vi "Initialize Parameter File.vi"(6 "File type":enum16{"INI"}(ring), 8 "error in (no error)":errorcluster, 9 "create file if necessary (T)":bool=TRUE, 10 "configuration file path (blank opens dialog)":path, 11 "CD Parameter Manager in":refnum<class "CD Parameter Manager.lvclass">) -> (0 "error out":errorcluster, 3 "CD Parameter Manager out":refnum<class "CD Parameter Manager.lvclass">)   [LabVIEW 2019, in "CD Parameter Manager API.lvlib" / "CD Parameter Manager.lvclass"]
uses:
  CD Parameter Manager.lvclass
  Parameter INI File/Parameter INI File.lvclass
  C:/Repositories/UI-Control-Initializer-API/Source/Parameter Generic File/Parameter Generic File.lvclass
  CD Parameter Manager.lvclass/CD Parameter Manager.ctl
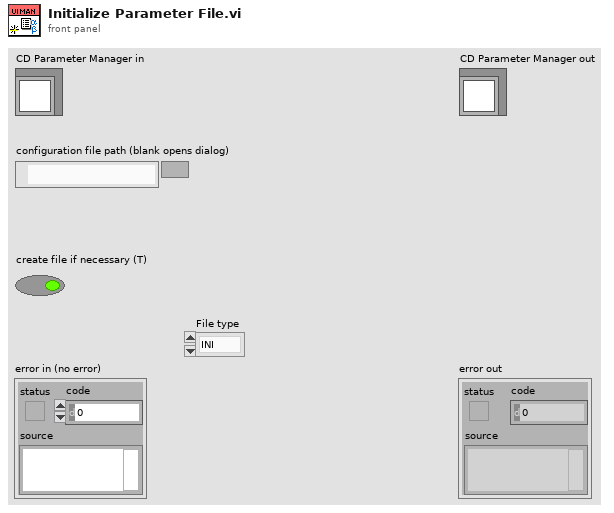
[diagram p1: front panel]
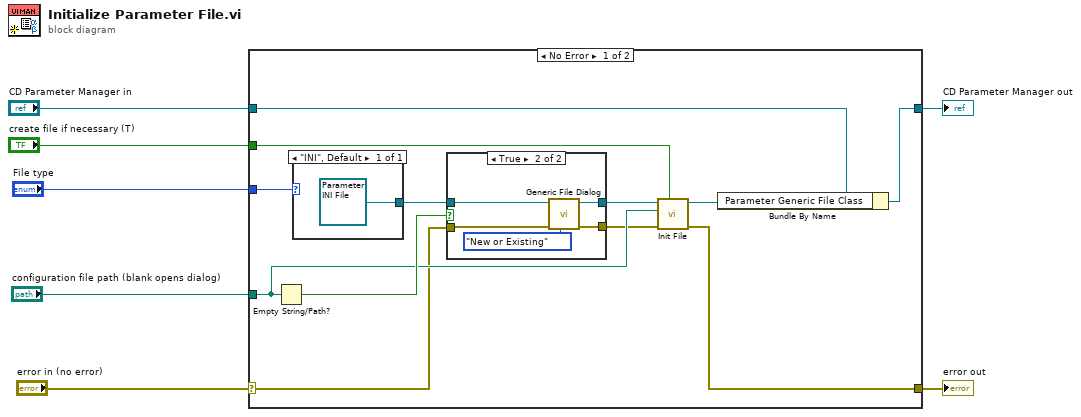
[diagram p0: block diagram]
diagram:
  n1 = case shown="No Error" "error in (no error)" {
    selector: "error in (no error)" -> [w14 w29]
    tunnel: [w10 w29] -> w6
    tunnel: [w8 w28] -> w4
    tunnel: "CD Parameter Manager in" -> [w13 w28]
    tunnel: "File type" -> [w19 _]
    tunnel: "configuration file path (blank opens dialog)" -> [w15 _]
    tunnel: "create file if necessary (T)" -> [w9 _]
    frame No Error {
      n2 = Empty String/Path?(string/path=w15) -> (empty?=w18:bool)
      n3 = case shown="\"INI\", Default" w19 {
        tunnel: [refnum<class "Parameter INI File.lvclass"> refnum ("CD Parameter Manager API.lvlib:Parameter INI File.lvclass")] -> w17
        frame "INI", Default {
        }
      }
      n4 = case shown="True" w18 {
        tunnel: w17 -> [w21 w26]
        tunnel: [w21 w25] -> w16
        tunnel: w14 -> [w20 w24]
        tunnel: [w20 w23] -> w11
        frame False {
        }
        frame True {
          n5 = call-dynamic "Generic File Dialog.vi"("Selection mode"=enum16{"New", "Existing", "New or Existing"}."New or Existing", "error in (no error)"=w24, "Parameter INI File in"=w26) -> ("error out"=w23:errorcluster, "Parameter INI File out"=w25:refnum<class "Parameter INI File.lvclass">)  [unwired: 7 in]
        }
      }
      n6 = call-dynamic "Init File.vi"("create file if necessary (T)"=w9, "error in (no error)"=w11, "configuration file path"=w15, "Parameter INI File in"=w16) -> ("error out"=w10:errorcluster, "Parameter INI File out"=w12:refnum<class "Parameter INI File.lvclass">)  [unwired: 6 in]
      n7 = Bundle By Name(cluster=w13, "Parameter Generic File Class"=w12) -> (w8:refnum<class "CD Parameter Manager.lvclass">)
    }
    frame Error {
    }
  }
  "error out" <- w6
  "CD Parameter Manager out" <- w4
